vi "Read Output.vi"(8 "error in (no error)":errorcluster, 11 "VISA resource name":refnum<visa-resource-name>) -> (0 "error out":errorcluster, 1 "Actual Current Level (amperes)":dbl, 2 "Actual Voltage Level (volts)":dbl, 3 "VISA resource name out":refnum<visa-resource-name>)   [LabVIEW 2018, in "XP Power PLS600.lvlib"]
doc: "Returns the actual voltage level and actual current level of the power supply output."
uses:
  XP Power PLS600.lvlib
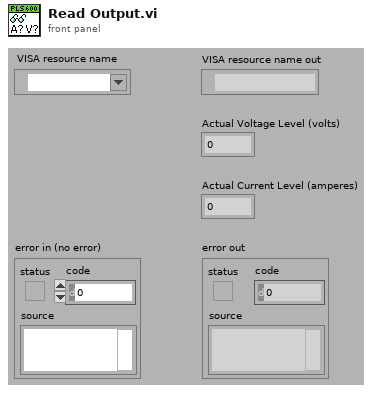
[diagram p1: front panel]
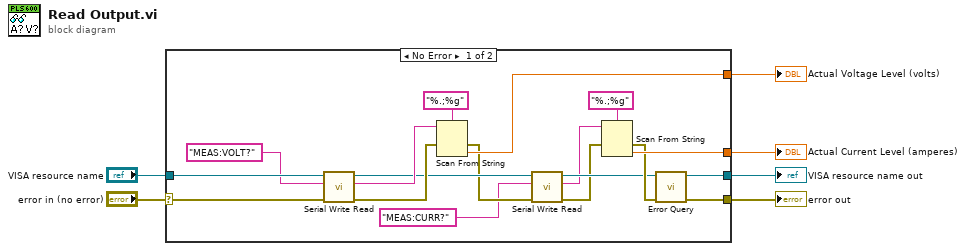
[diagram p0: block diagram]
diagram:
  n1 = case shown="No Error" "error in (no error)" {
    selector: "error in (no error)" -> [w7 w26]
    tunnel: [w24 w25] -> w6
    tunnel: [w23 w26] -> w5
    tunnel: [w21 _] -> w4
    tunnel: [w19 _] -> w3
    tunnel: "VISA resource name" -> [w17 w25]
    frame No Error {
      n2 = call "Serial Write Read.vi"("error in (no error)"=w7, "Write Buffer"="MEAS:VOLT?", "VISA resource name"=w17) -> ("error out"=w14:errorcluster, "Read Buffer"=w15:string, "VISA resource name out"=w13:refnum<visa-resource-name>)  [unwired: 6 in]
      n3 = Scan From String(format string="%.;%g", input string=w15, error in=w14) -> (error out=w9:errorcluster, output 1=w21:dbl)  [unwired: 2 in, 2 out]
      n4 = call "Serial Write Read.vi"("error in (no error)"=w9, "Write Buffer"="MEAS:CURR?", "VISA resource name"=w13) -> ("error out"=w10:errorcluster, "Read Buffer"=w11:string, "VISA resource name out"=w12:refnum<visa-resource-name>)  [unwired: 6 in]
      n5 = Scan From String(format string="%.;%g", input string=w11, error in=w10) -> (error out=w18:errorcluster, output 1=w19:dbl)  [unwired: 2 in, 2 out]
      n6 = call "Error Query.vi"("error in (no error)"=w18, "VISA resource name"=w12) -> ("error out"=w23:errorcluster, "VISA resource name out"=w24:refnum<visa-resource-name>)  [unwired: 6 in, 2 out]
    }
    frame Error {
    }
  }
  "VISA resource name out" <- w6
  "error out" <- w5
  "Actual Voltage Level (volts)" <- w4
  "Actual Current Level (amperes)" <- w3
